vi "Read Parameters.vi"(8 "error in (no error)":errorcluster, 11 "Data in":T1 {"#Bands" min=3 max=6 step=1}) -> (0 "error out":errorcluster, 3 "Data out":T1 {"#Bands" min=3 max=6 step=1})   [LabVIEW 2018]
uses:
  Data--cluster.ctl
  Digit--enum.ctl
  Multiplier--enum.ctl
  Tolerance--enum.ctl
  Temp Coeficient--enum.ctl
  E-Series Reader/Series Data--cluster.ctl
  In Low Series--cluster.ctl
  In Mid-High Series--cluster.ctl
  Number of Bands--number.ctl
  E-Series Reader/E-Series Reader.lvlib
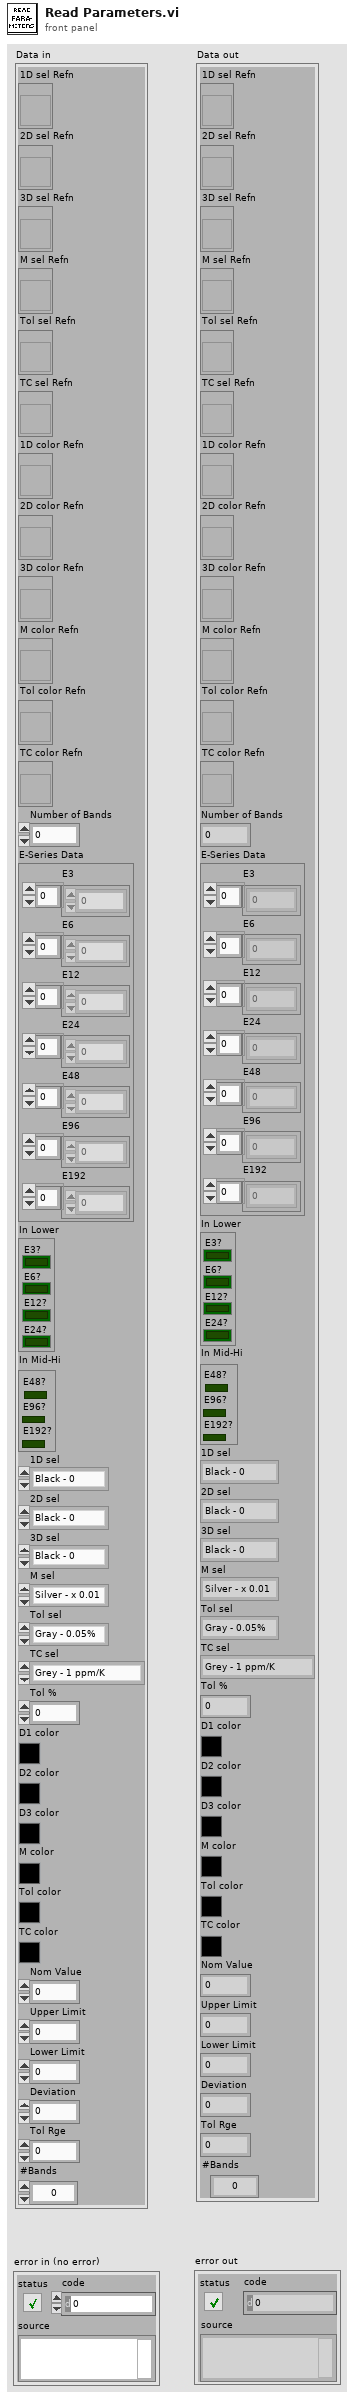
[diagram p1: front panel]
types:
  T1 = typedef "Data--cluster.ctl" = cluster{"1D sel Refn":refnum<vi>, "2D sel Refn":refnum<vi>, "3D sel Refn":refnum<vi>, "M sel Refn":refnum<vi>, "Tol sel Refn":refnum<vi>, "TC sel Refn":refnum<vi>, "1D color Refn":refnum<vi>, "2D color Refn":refnum<vi>, "3D color Refn":refnum<vi>, "M color Refn":refnum<vi>, "Tol color Refn":refnum<vi>, "TC color Refn":refnum<vi>, "Number of Bands":u8, "E-Series Data":T2, "In Lower":T3, "In Mid-Hi":T4, "1D sel":T5, "2D sel":T5, "3D sel":T5, "M sel":T6, "Tol sel":T7, "TC sel":T8, "Tol %":dbl, "D1 color":u32, "D2 color":u32, "D3 color":u32, "M color":u32, "Tol color":u32, "TC color":u32, "Nom Value":dbl, "Upper Limit":dbl, "Lower Limit":dbl, "Deviation":dbl, "Tol Rge":dbl, "#Bands":T9}
  T2 = typedef "E-Series Reader.lvlib/series data--cluster.ctl" = cluster{"E3":u16[], "E6":u16[], "E12":u16[], "E24":u16[], "E48":u16[], "E96":u16[], "E192":u16[]}
  T3 = typedef "In low series--cluster.ctl" = cluster{"E3?":bool, "E6?":bool, "E12?":bool, "E24?":bool}
  T4 = typedef "In mid-high series--cluster.ctl" = cluster{"E48?":bool, "E96?":bool, "E192?":bool}
  T5 = typedef "digit--enum.ctl" = enum16{"Black - 0", "Brown - 1", "Red - 2", "Orange - 3", "Yellow - 4", "Green - 5", "Blue - 6", "Violet - 7", "Grey - 8", "White - 9"}
  T6 = typedef "multiplier--enum.ctl" = enum16{"Silver - x 0.01", "Gold - x 0.1 ", "Black - x 1", "Brown - x 10", "Red - x 100", "Orange - x 1k", "Yellow - x 10k", "Green - 100k", "Blue - x 1M", "Violet - x10 M", "Grey - x 100M", "White - x 1G"}
  T7 = typedef "tolerance--enum.ctl" = enum16{"Gray - 0.05%", "Violet - 0.1%", "Blue - 0.25%", "Green - 0.5%", "Brown - 1%", "Red - 2%", "Gold - 5%", "Silver - 10%", "None - 20%"}
  T8 = typedef "temp coeficient--enum.ctl" = enum16{"Grey - 1 ppm/K", "Violet - 5 ppm/K", "Blue - 10 ppm/K", "Green - 20 ppm/K", "Yellow - 25 ppm/K", "Orange - 15 ppm/K", "Red - 50 ppm/K", "Brown - 100 ppm/K", "Black - 250 ppm/K"}
  T9 = typedef "Number of Bands--number.ctl" = u8
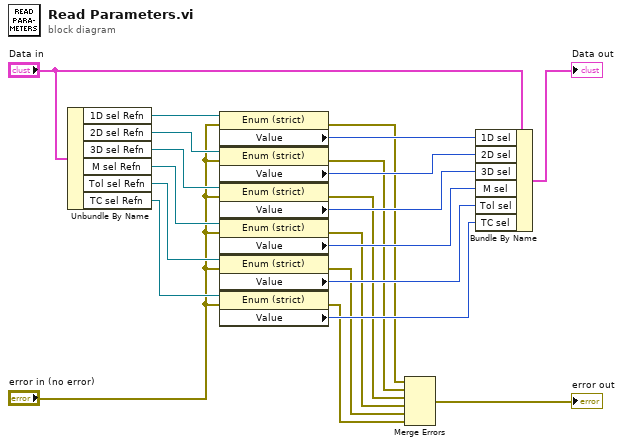
[diagram p0: block diagram]
diagram:
  n1 = Unbundle By Name("Data in") -> ("1D sel Refn"=w9:refnum<vi>, "2D sel Refn"=w10:refnum<vi>, "3D sel Refn"=w11:refnum<vi>, "M sel Refn"=w12:refnum<vi>, "Tol sel Refn"=w13:refnum<vi>, "TC sel Refn"=w14:refnum<vi>)
  n2 = property class="Enum (strict)"(reference=w9, error in="error in (no error)") -> (error out=w2:errorcluster, "Value"=w17:T5)  [unwired: 1 out]
  n3 = property class="Enum (strict)"(reference=w10, error in="error in (no error)") -> (error out=w3:errorcluster, "Value"=w18:T5)  [unwired: 1 out]
  n4 = property class="Enum (strict)"(reference=w11, error in="error in (no error)") -> (error out=w4:errorcluster, "Value"=w19:T5)  [unwired: 1 out]
  n5 = property class="Enum (strict)"(reference=w12, error in="error in (no error)") -> (error out=w5:errorcluster, "Value"=w20:T6)  [unwired: 1 out]
  n6 = property class="Enum (strict)"(reference=w13, error in="error in (no error)") -> (error out=w6:errorcluster, "Value"=w21:T7)  [unwired: 1 out]
  n7 = property class="Enum (strict)"(reference=w14, error in="error in (no error)") -> (error out=w7:errorcluster, "Value"=w22:T8)  [unwired: 1 out]
  n8 = Merge Errors(w2, w3, w4, w5, w6, w7) -> (→"error out":errorcluster)
  n9 = Bundle By Name(cluster="Data in", "1D sel"=w17, "2D sel"=w18, "3D sel"=w19, "M sel"=w20, "Tol sel"=w21, "TC sel"=w22) -> (→"Data out":T1)
